vi "Configure Trigger Core.vi"(8 "error in (no error)":errorcluster, 9 "trigger holdoff (500.0 E-9 s)":dbl[unit]=5e-07 format="%^.2e", 10 "trigger type (Edge)":i32(ring)=1 items=["Edge"=1, "TV"=5, "Runt"=3, "Glitch"=4, "Width"=2, "AC Line"=7, "Immediate"=6], 11 "IVI_Scope in":refnum<class "IVI_Scope.lvclass">) -> (0 "error out":errorcluster, 3 "IVI_Scope out":refnum<class "IVI_Scope.lvclass">)   [LabVIEW 2016, in "IVI_Scope.lvlib" / "IVI_Scope.lvclass"]
doc: "This VI configures the common properties of the trigger subsystem. These properties are the trigger type and holdoff.\nWhen you call IviScope Read Waveform, IviScope Read Waveform Measurement [WM], IviScope Read Min Max Waveform [MmW], or IviScope Initiate Acquisition, the oscilloscope waits for a trigger. You specify the type of trigger for which the oscilloscope waits with the Trigger Type parameter.\nIf the oscilloscope requires multiple waveform acquisitions to build a complete waveform, it waits for the length of time you specify with the Holdoff parameter to elapse since the previous trigger. The oscilloscope then waits for the next trigger. Once the oscilloscope acquires a complete waveform, it returns to the Idle state."
uses:
  IVI_Scope.lvclass
  IVI_Scope.lvclass/IVI_Scope.ctl
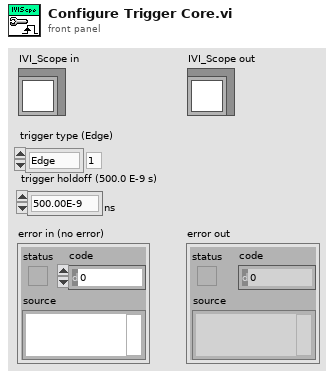
[diagram p1: front panel]
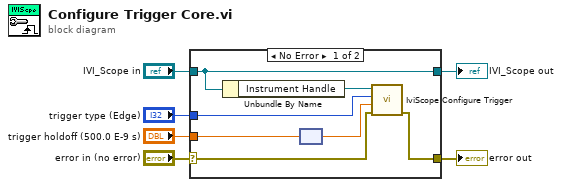
[diagram p0: block diagram]
diagram:
  n1 = case shown="No Error" "error in (no error)" {
    selector: "error in (no error)" -> [w10 w15]
    tunnel: [w9 w15] -> w5
    tunnel: [w13 w14] -> w3
    tunnel: "IVI_Scope in" -> [w13 w14]
    tunnel: "trigger type (Edge)" -> [w11 _]
    tunnel: "trigger holdoff (500.0 E-9 s)" -> [w8 _]
    frame No Error {
      n2 = Unbundle By Name(w13) -> ("Instrument Handle"=w12:refnum<k15>)
      n3 = node(w8) -> (w7:dbl)
      n4 = call <vilib>:"IviScope Configure Trigger.vi"("error in (no error)"=w10, "trigger holdoff (500.0 E-9 s)"=w7, "trigger type (Edge)"=w11, "instrument handle"=w12) -> ("error out"=w9:errorcluster)  [unwired: 6 in, 1 out]
    }
    frame Error {
    }
  }
  "error out" <- w5
  "IVI_Scope out" <- w3
